vi "Set Resource.vi"(8 "error in (no error)":errorcluster, 10 "Resource":refnum<class "DeployResource.lvclass">, 11 "Device in":refnum<class "Device.lvclass">) -> (0 "error out":errorcluster, 3 "Device out":refnum<class "Device.lvclass">)   [LabVIEW 2020, in "PicoG-Core.lvlib" / "Device.lvclass"]
uses:
  Device.lvclass
  DeployResource/DeployResource.lvclass
  Device.lvclass/Device.ctl
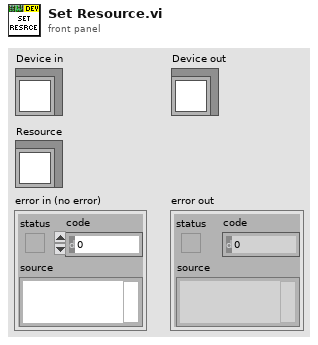
[diagram p1: front panel]
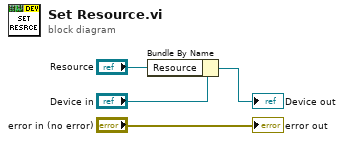
[diagram p0: block diagram]
diagram:
  n1 = Bundle By Name(cluster="Device in", "Resource"="Resource") -> (→"Device out":refnum<class "Device.lvclass">)
  "error out" <- "error in (no error)"
